vi "beep_pc_speaker_lv821.vi"   [LabVIEW 2012]
doc: "Causes the system to issue an audible tone."
uses:
  KERNEL32.DLL
panel:
  # "See block diagram for instructions."
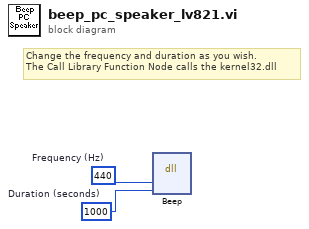
[diagram p0: block diagram]
diagram:
  w1 = 440  # Frequency (Hz)
  w2 = 1000  # Duration (seconds)
  # "Change the frequency and duration as you wish.\nThe Call Library Function Node calls the kernel32.dll"
  n1 = dll-call lib="KERNEL32.DLL" fn="Beep"(w1, w2) -> ()  [unwired: 6 in, 2 out]
